vi "DG535ErrorHandler.vi"(8 "error in":errorcluster, 11 "VISA resource name":refnum<visa-resource-name>) -> (0 "error out":errorcluster, 2 "error found":bool, 3 "duplicate VISA resource":refnum<visa-resource-name>)   [LabVIEW 2012, in "SRS_DG535_Lib.lvlib"]
doc: "This support subVI queries the instrument's error status bits which reports an execution error .\n ERROR FOUND is set to TRUE when an out of range parameter or a delay linkage error causes an execution error . \n This subVI is used in the function subVIs after setting some or all of the instrument's functions .\n The status of ERROR FOUND is then used in the function subVIs to report an error for the parameter that caused it ."
uses:
  SRS_DG535_Lib.lvlib
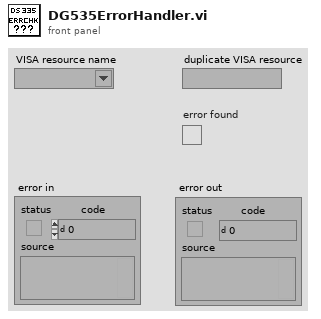
[diagram p1: front panel]
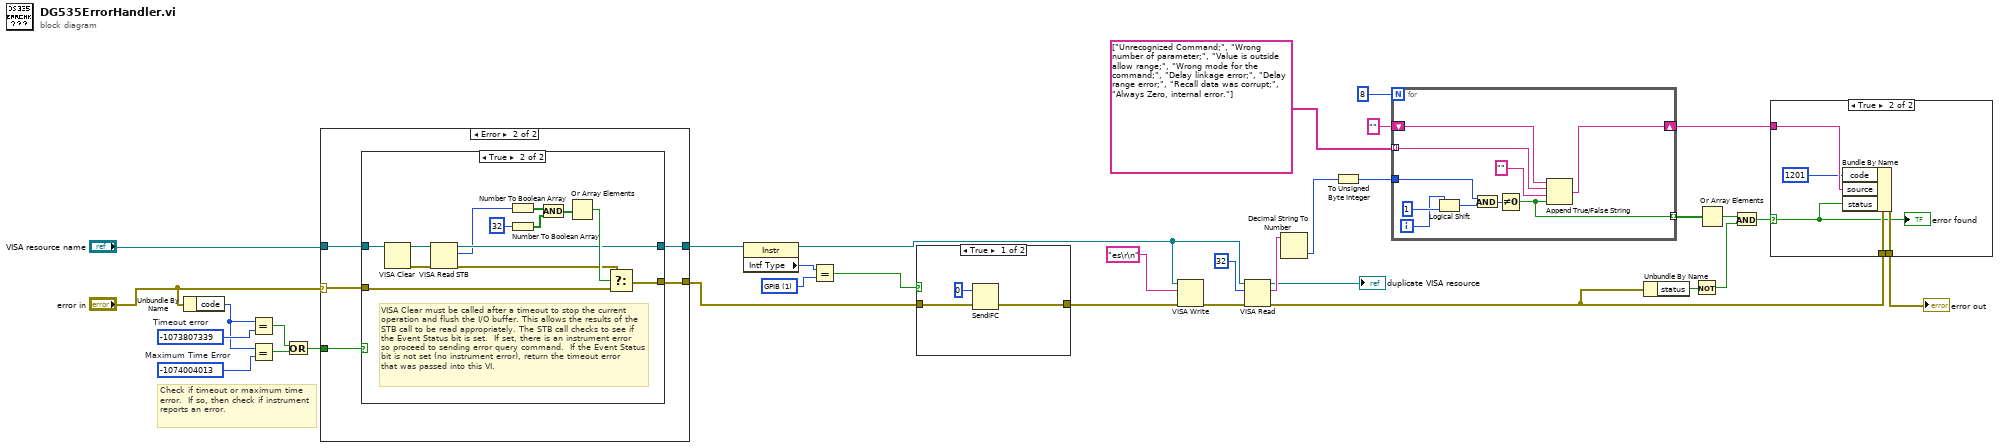
[diagram p0: block diagram]
diagram:
  w8 = -1074004013  # Maximum Time Error
  w10 = -1073807339  # Timeout error
  w13 = u16 1 items=["GPIB"=1, "VXI"=2, "GPIB-VXI"=3, "Serial"=4, "PXI"=5, "TCPIP"=6, "USB"=7, "FireWire"=9] ("Interface Information:Interface Type")
  # "Check if timeout or maximum time error.  If so, then check if instrument reports an error."
  n1 = Unbundle By Name("error in") -> ("code"=w9:i32)
  n2 = Equal?(x=w9, y=w10) -> (x = y?=w6:bool)
  n3 = Equal?(x=w9, y=w8) -> (x = y?=w7:bool)
  n4 = Or(x=w6, y=w7) -> (x .or. y?=w5:bool)
  n5 = case shown="Error" "error in" {
    selector: "error in" -> [w34 w38]
    tunnel: "VISA resource name" -> [w35 w40]
    tunnel: [w35 w39] -> w2
    tunnel: [w34 w37] -> w1
    tunnel: w5 -> [_ w36]
    frame No Error {
    }
    frame Error {
      n6 = case shown="True" w36 {
        tunnel: w40 -> [w42 w48]
        tunnel: [w42 w45] -> w39
        tunnel: w38 -> [w41 w51]
        tunnel: [w41 w50] -> w37
        frame False {
          # "Error code not a timeout, so best to pass on to user."
        }
        frame True {
          # "VISA Clear must be called after a timeout to stop the current operation and flush the I/O buffer. This allows the results of the  STB call to be read appropriately. The STB call checks to see if the Event Status bit is set.  If set, there is an instrument error so proceed to sending error query command.  If the Event Status bit is not set (no instrument error), return the timeout error that was passed into this VI."
          n7 = VISA Clear(VISA resource name=w48) -> (VISA resource name out=w47:refnum<visa-resource-name>, error out=w46:errorcluster)  [unwired: 1 in]
          n8 = VISA Read STB(8:w46, 11:w47) -> (0:w44:errorcluster, 2:w43:u16, 3:w45:refnum<visa-resource-name>)
          n9 = Number To Boolean Array(number=w43) -> (Boolean array=w52:bool[])
          n10 = Number To Boolean Array(number=32) -> (Boolean array=w54:bool[])
          n11 = And(x=w52, y=w54) -> (x .and. y?=w53:bool[])
          n12 = Or Array Elements(Boolean array=w53) -> (logical OR=w49:bool)
          n13 = Select(t=w44, s=w49, f=w51) -> (s? t:f=w50:errorcluster)
        }
      }
    }
  }
  n14 = property class="Instr"(reference=w2) -> (reference out=w14:refnum<visa-resource-name>, "Intf Type"=w12:u16)  [unwired: 1 in, 1 out]
  n15 = Equal?(x=w12, y=w13) -> (x = y?=w11:bool)
  n16 = case shown="True" w11 {
    tunnel: w1 -> [w57 w59]
    tunnel: [w56 w59] -> w28
    frame True {
      n17 = SendIFC(2:w57, 3:0) -> (0:w56:errorcluster)  [unwired: 1 out]
    }
    frame False {
    }
  }
  n18 = VISA Write(VISA resource name=w14, write buffer="es\r\n" ("command string"), error in (no error)=w28) -> (error out=w27:errorcluster)  [unwired: 2 out]
  n19 = VISA Read(VISA resource name=w14, byte count=u32 32, error in (no error)=w27) -> (VISA resource name out=→"duplicate VISA resource":refnum<visa-resource-name>, read buffer=w26:string, error out=w33:errorcluster)  [unwired: 1 out]
  n20 = Decimal String To Number(string=w26) -> (number=w20:i32)  [unwired: 2 in, 1 out]
  n21 = To Unsigned Byte Integer(number=w20) -> (unsigned 8bit integer=w23:u8)
  n22 = for {
    N: 8 -> [_]
    tunnel: w23 -> [w66]
    shift-right: [w63] -> w16
    shift-left: "" ("output string") -> [w64]
    tunnel: string[] ["Unrecognized Command;", "Wrong number of parameter;", "Value is outside allow range;", "Wrong mode for the command;", "Delay linkage error;", "Delay range error;", "Recall data was corrupt;", "Always Zero, internal error."] -> [w62] mode=indexing
    tunnel: [w60] -> w19 mode=indexing
    i -> [w68]
    n23 = Logical Shift(y=w68, x=u8 1 ("y")) -> (x << y=w67:u8)
    n24 = And(x=w66, y=w67) -> (x .and. y?=w65:u8)
    n25 = Not Equal To 0?(x=w65) -> (x != 0?=w60:bool)
    n26 = Append True/False String(1:w60, 2:"" ("false string"), 3:w62, 4:w64) -> (0:w63:string)
  }
  n27 = Unbundle By Name(w33) -> ("status"=w30:bool)
  n28 = Not(x=w30) -> (.not. x?=w29:bool)
  n29 = Or Array Elements(Boolean array=w19) -> (logical OR=w18:bool)
  n30 = And(x=w18, y=w29) -> (x .and. y?=w15:bool)
  n31 = case shown="True" w15 {
    selector: w15 -> [_ w71]
    tunnel: w33 -> [w70 w75]
    tunnel: [w70 w74] -> w17
    tunnel: w16 -> [_ w73]
    frame False {
    }
    frame True {
      n32 = Bundle By Name(cluster=w75, "code"=1201, "source"=w73, "status"=w71) -> (w74:errorcluster)
      "error found" <- w71
    }
  }
  "error out" <- w17
